vi "ICR_Start_Timer.vi"(8 "error in (no error)":errorcluster, 11 "QMH ICR Cluster":T1) -> (0 "error out":errorcluster, 3 "QMH ICR Cluster":T1)   [LabVIEW 2024]
doc: "This VI inits a waveform generation session for both HSDIO 6541 and AWG 5421. This is a basic example that shows how to setup the board in order to generate waveforms according to a script. \n\n1. Initialize for a generation session.\n2. Assign specified channels in Channel List for dynamic operation : all = \"\" (default)\n3. Sets the Idle State for when the generation has completed : NO !!\n4. Configure the Sample clock to use the onboard clock, and configure the clock rate.\n5. Set generation mode to Scripted.\n6. Configure the Script Trigger : change to Digital Edge if waiting for an external\n trigger, and link Rising Edge and source trigger commands.\n Use PFI0 with SMB wired to the board, or any PFIxx if connected to accessory."
uses:
  controls/QMH_ICR_Cluster.ctl
  controls/HARDWARE_Resources.ctl
  controls/PROCESSING_Inputs.ctl
  controls/LOOPS_Inputs.ctl
  controls/OPO_Inputs.ctl
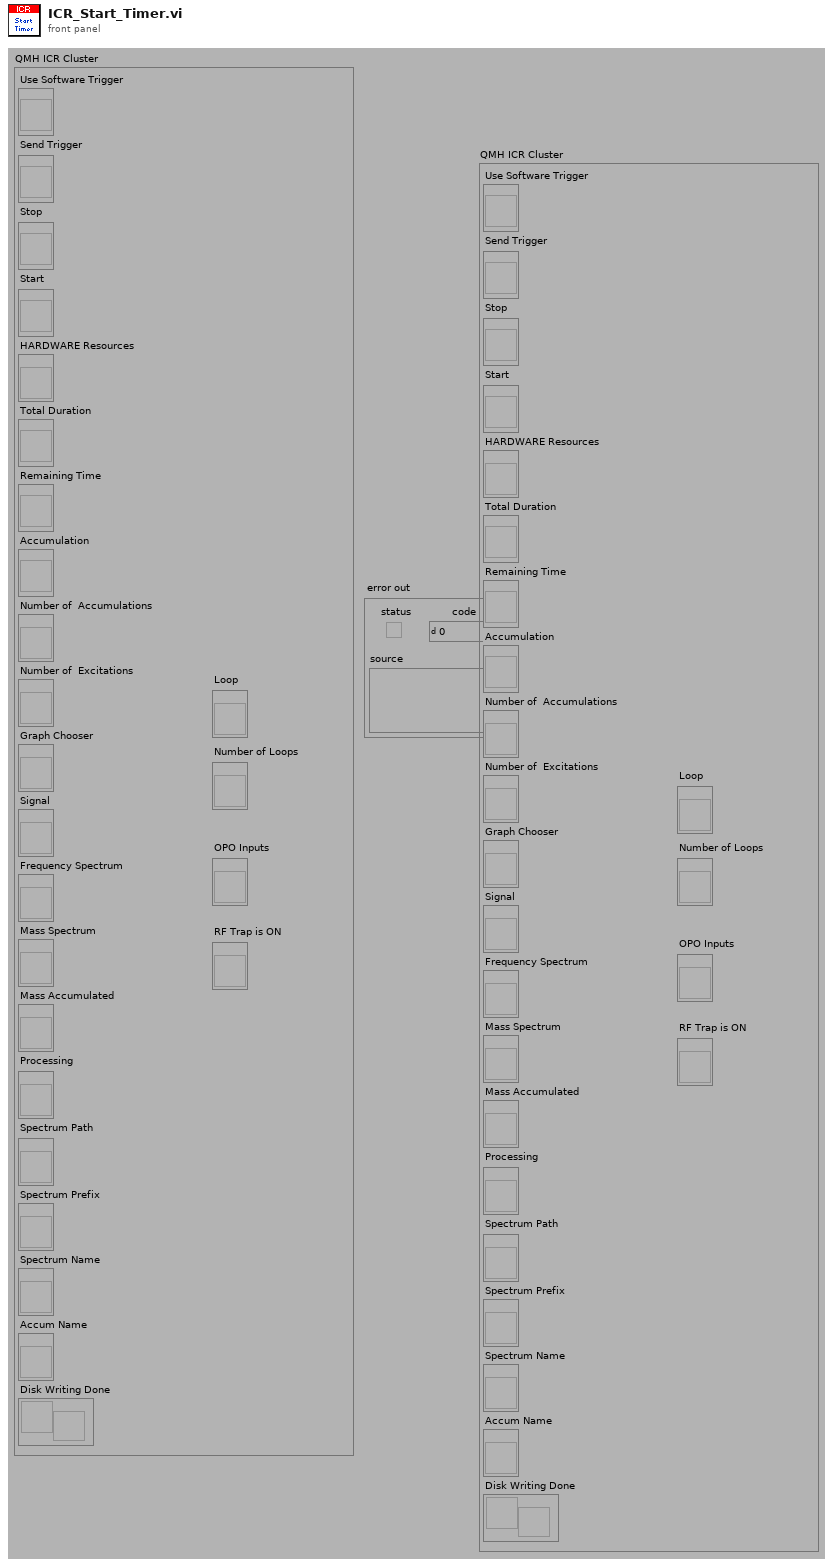
[diagram p1: front panel]
types:
  T1 = typedef "QMH_ICR_Cluster.ctl" = cluster{"Use Software Trigger":refnum<vi>, "Send Trigger":refnum<vi>, "Stop":refnum<vi>, "Start":refnum<vi>, "HARDWARE Resources":refnum<vi>, "Total Duration":refnum<vi>, "Remaining Time":refnum<vi>, "Accumulation":refnum<vi>, "Number of  Accumulations":refnum<vi>, "Number of  Excitations":refnum<vi>, "Graph Chooser":refnum<vi>, "Signal":refnum<vi>, "Frequency Spectrum":refnum<vi>, "Mass Spectrum":refnum<vi>, "Mass Accumulated":refnum<vi>, "Processing":refnum<vi>, "Spectrum Path":refnum<vi>, "Spectrum Prefix":refnum<vi>, "Spectrum Name":refnum<vi>, "Accum Name":refnum<vi>, "Disk Writing Done":refnum<notifier>, "Loop":refnum<vi>, "Number of Loops":refnum<vi>, "OPO Inputs":refnum<vi>, "RF Trap is ON":refnum<vi>}
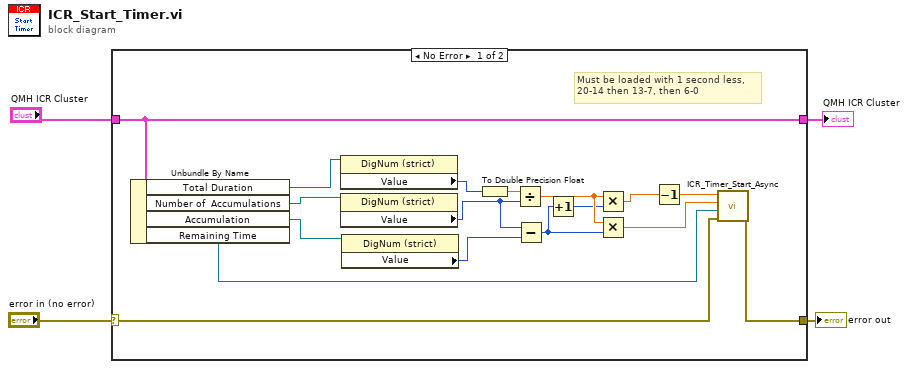
[diagram p0: block diagram]
diagram:
  n1 = case shown="No Error" "error in (no error)" {
    selector: "error in (no error)" -> [w19 w23]
    tunnel: [w18 w23] -> w4
    tunnel: "QMH ICR Cluster" -> [w21 w22]
    tunnel: [w21 w22] -> w1
    frame No Error {
      # "Must be loaded with 1 second less,\n20-14 then 13-7, then 6-0"
      n2 = Unbundle By Name(w21) -> ("Total Duration"=w20:refnum<vi>, "Number of  Accumulations"=w15:refnum<vi>, "Accumulation"=w14:refnum<vi>, "Remaining Time"=w7:refnum<vi>)
      n3 = property class="DigNum (strict)"(reference=w20) -> ("Value"=w17:i32)  [unwired: 1 in, 2 out]
      n4 = property class="DigNum (strict)"(reference=w15) -> ("Value"=w12:i16)  [unwired: 1 in, 2 out]
      n5 = property class="DigNum (strict)"(reference=w14) -> ("Value"=w13:i16)  [unwired: 1 in, 2 out]
      n6 = To Double Precision Float(number=w17) -> (double precision float=w16:dbl)
      n7 = Divide(x=w16, y=w12) -> (x/y=w10:dbl)
      n8 = Subtract(x=w12, y=w13) -> (x-y=w9:i16)
      n9 = Increment(x=w9) -> (x+1=w6:i16)
      n10 = Multiply(x=w10, y=w6) -> (x*y=w11:dbl)
      n11 = Multiply(x=w10, y=w9) -> (x*y=w8:dbl)
      n12 = Decrement(x=w11) -> (x-1=w5:dbl)
      n13 = call "ICR_Timer_Start_Async.vi"("Seconds"=w5, "Last Seconds"=w8, "Refnum Ch"=w7, "error in (no error)"=w19) -> ("error out"=w18:errorcluster)  [unwired: 6 in]
    }
    frame Error {
    }
  }
  "error out" <- w4
  "QMH ICR Cluster" <- w1
